vi "Write CSV File.vi"(0 "Refnum In":refnum<file>, 7 "Data":string[](array[string]), 11 "Error In":errorcluster) -> (4 "Refnum Out":refnum<file>, 15 "Error Out":errorcluster)   [LabVIEW 2016]
doc: "This vi writes a 1D string array to a csv file. It is programmed to allways append to the end of the csv file. This string array is normally going to be data parsed from ERDs, or data obtained from DAQ, formated to string data type and added to a 1D array. The array order should match order of header created for csv file.\n\nThe refnum out will need to be closed elsewere in main VI using Close File.vi"
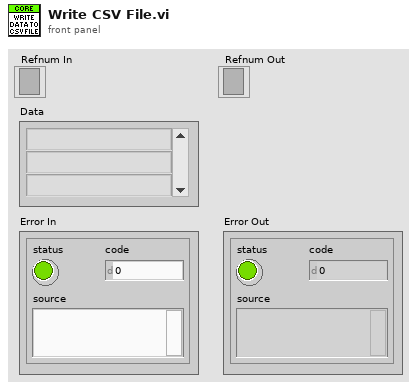
[diagram p1: front panel]
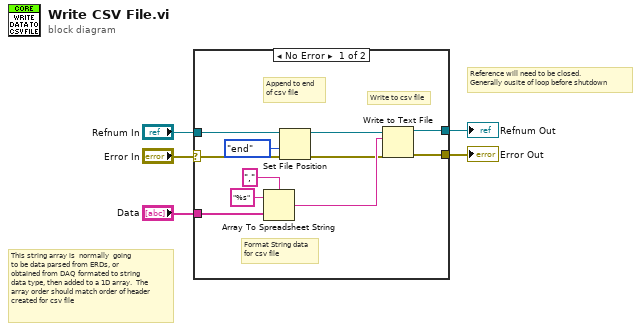
[diagram p0: block diagram]
diagram:
  # "Reference will need to be closed.\nGenerally ousite of loop before shutdown"
  # "This string array is  normally  going\nto be data parsed from ERDs, or\nobtained from DAQ formated to string\ndata type, then added to a 1D array.  The \narray order should match order of header\ncreated for csv file"
  n1 = case shown="No Error" "Error In" {
    selector: "Error In" -> [w9 w18]
    tunnel: [w15 w17] -> w4
    tunnel: "Refnum In" -> [w13 w17]
    tunnel: [w10 w18] -> w3
    tunnel: "Data" -> [w6 _]
    frame No Error {
      # "Write to csv file"
      # "Append to end\nof csv file"
      # "Format String data\nfor csv file"
      n2 = Array To Spreadsheet String(delimiter (Tab)=",", array=w6, 3:"%s" ("format string")) -> (spreadsheet string=w16:string)
      n3 = Set File Position(refnum=w13, from (0:start)=enum16{"start", "end", "current"}."end", error in=w9) -> (refnum out=w12:refnum<file>, error out=w11:errorcluster)  [unwired: 1 in]
      n4 = Write to Text File(file (use dialog)=w12, text=w16, error in=w11) -> (refnum out=w15:refnum<file>, error out=w10:errorcluster)  [unwired: 1 in, 1 out]
    }
    frame Error {
    }
  }
  "Error Out" <- w3
  "Refnum Out" <- w4
